vi "STAT2 Decode Analog data from Tensionsub Node.vi"(9 "Temperature base conversion factor":u16=128, 10 "Tension Sub":T1 {"sys register" format="%04x"}) -> (2 "Node Analog value":dbl[](array[numeric]), 3 "Temperature":dbl)   [LabVIEW 2011]
uses:
  LEINmaster/Nodes/tensionsub stat2.ctl
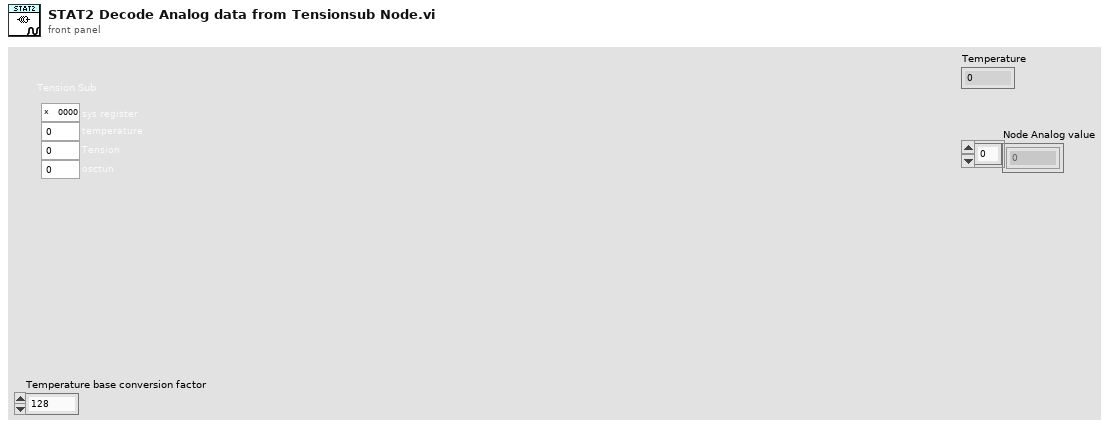
[diagram p1: front panel]
types:
  T1 = typedef "tensionsub stat2.ctl" = cluster{"sys register":u16, "temperature":u16, "Tension":i16, "osctun":u8}
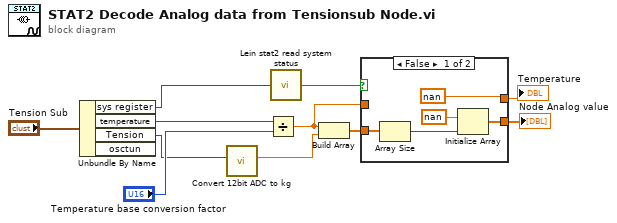
[diagram p0: block diagram]
diagram:
  n1 = Unbundle By Name("Tension Sub") -> ("sys register"=w6:u16, "temperature"=w11:u16, "Tension"=w3:i16)  [unwired: 1 out]
  n2 = call "Convert 12bit ADC to kg.vi"("ADC"=w3) -> ("output"=w2:dbl)  [unwired: 10 in]
  n3 = Divide(x=w11, y="Temperature base conversion factor") -> (x/y=w5:dbl)
  n4 = call "Lein stat2 read system status.vi"("sys register"=w6) -> ("Connected"=w9:bool)  [unwired: 7 in, 7 out]
  n5 = Build Array(w5, w2) -> (w8:dbl[])
  n6 = case shown="False" w9 {
    tunnel: [w13 w18] -> w7
    tunnel: w8 -> [w16 w18]
    tunnel: [nan ("element") w17] -> w4
    tunnel: w5 -> [_ w17]
    frame False {
      n7 = Array Size(array=w16) -> (size(s)=w15:i32)
      n8 = Initialize Array(nan ("element"), w15) -> (w13:dbl[])
    }
    frame True {
    }
  }
  "Node Analog value" <- w7
  "Temperature" <- w4
